vi "working_interface_timing.vi"(10 "VISA resource name":refnum<visa-resource-name>="TRIG") -> (2 "data in delay generator":dbl[](array[numeric]) caption="delay array" min=0.0 max=2000.0 format="%05.2f")   [LabVIEW 2011]
panel:
  out "timing write":u32
  in  "time unit":enum16{"s", "ms", "us", "ns"}(ring)=enum."us"
  in  "resolution":i32=100
  in  "duration":dbl[](array[numeric]) min=0.0 format="%.3f"
  in  "start time":dbl[](array[numeric]) format="%.3f"
  out "Digital Waveform Graph":digitalwaveform(graph)
  in  "write data":bool
  in  "read delay data":bool
  in  "stop":bool
  # "timing values are only relative,\n the absolute values are given in the\ndelay array!!!\n\nt0 and t can not be written to the device, t0 is always 0\nand  t is always the longest time + 25ns. However, t is \nused to display how long the nozzle is open to give a real \nrepresentation in the diagram (and only there). \nYou can change that time to pretty much any value, \nbut the nozzle itself is not controlled through the labview\n software. You have to set the time manually at the \nnozzle driver and ideally you should then enter that time\nfor t as well!\n\ndelay array index:\n0 - t0 = nozzle start (TTL) = 0\n1 - nozzle duration\n2 - power AMP START\n3 - power AMP STOP\n4 - AWG START (TTL)\n5 - AWG STOP (NA)\n6 - SWITCH ON \n7 - SWITCH OFF\n8 - OSC START (TTL)\n9 - OSC STOP (NA)\n\nTTL -> tool starts on rising flank\nof signal, hence the falling flank \nand the duration are not important!"
  # "t0 is always 0"
  # "AWG must start after power AMP is on \nand while it is still on!"
  # "SWITCH must NOT switch ON before \npower AMP is off!"
  # "delay array index:\n0 - to = nozzle start (TTL) = 0\n1 - t = nozzle duration\n2 - A = power AMP START\n3 - B = power AMP STOP\n4 - C = AWG START (TTL)\n5 - D = AWG STOP (NA)\n6 - E = SWITCH ON \n7 - F = SWITCH OFF\n8 - G = OSC START (TTL)\n9 - H = OSC STOP (NA)\n\nTTL -> tool starts on rising flank\nof signal, hence the falling flank \nand the duration are not important!"
  # "the graph does not show the actual TTL signal for all signals. For those with negative polarity it shows the inverse of the signal \nit shows when everything is active"
  # "nozzle"
  # "power AMP"
  # "AWG"
  # "SWITCH"
  # "OSC"
  # "t0"
  # "t"
  # "A"
  # "B"
  # "C"
  # "D"
  # "E"
  # "F"
  # "G"
  # "H"
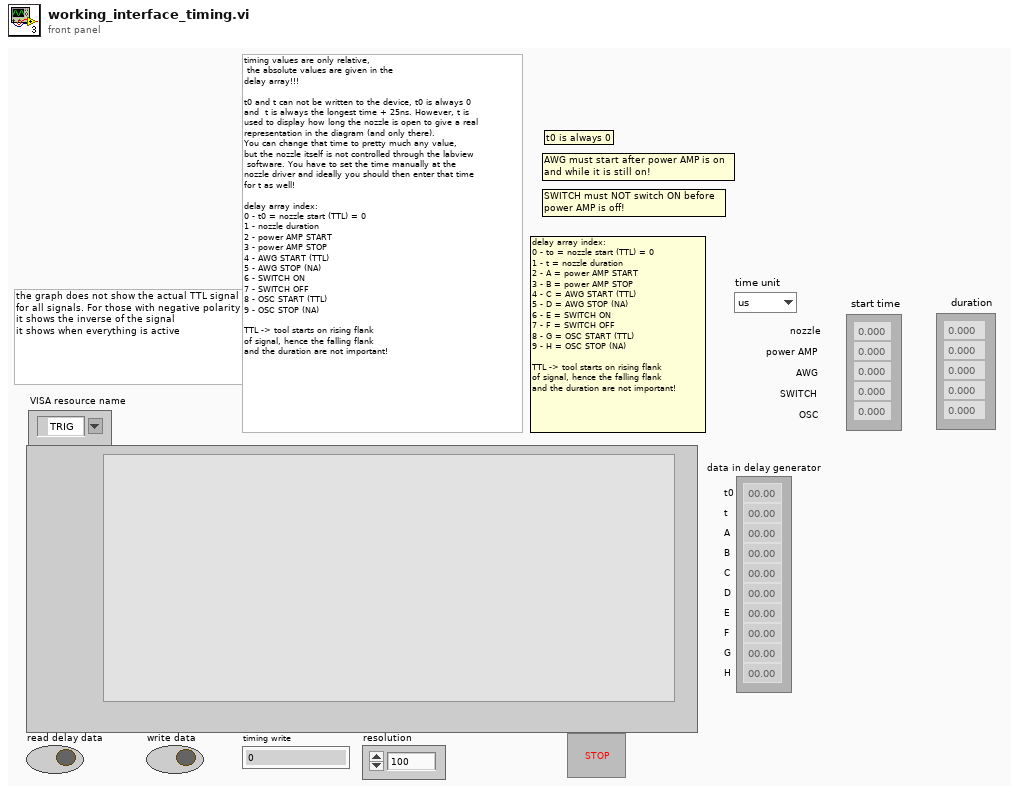
[diagram p1: front panel]
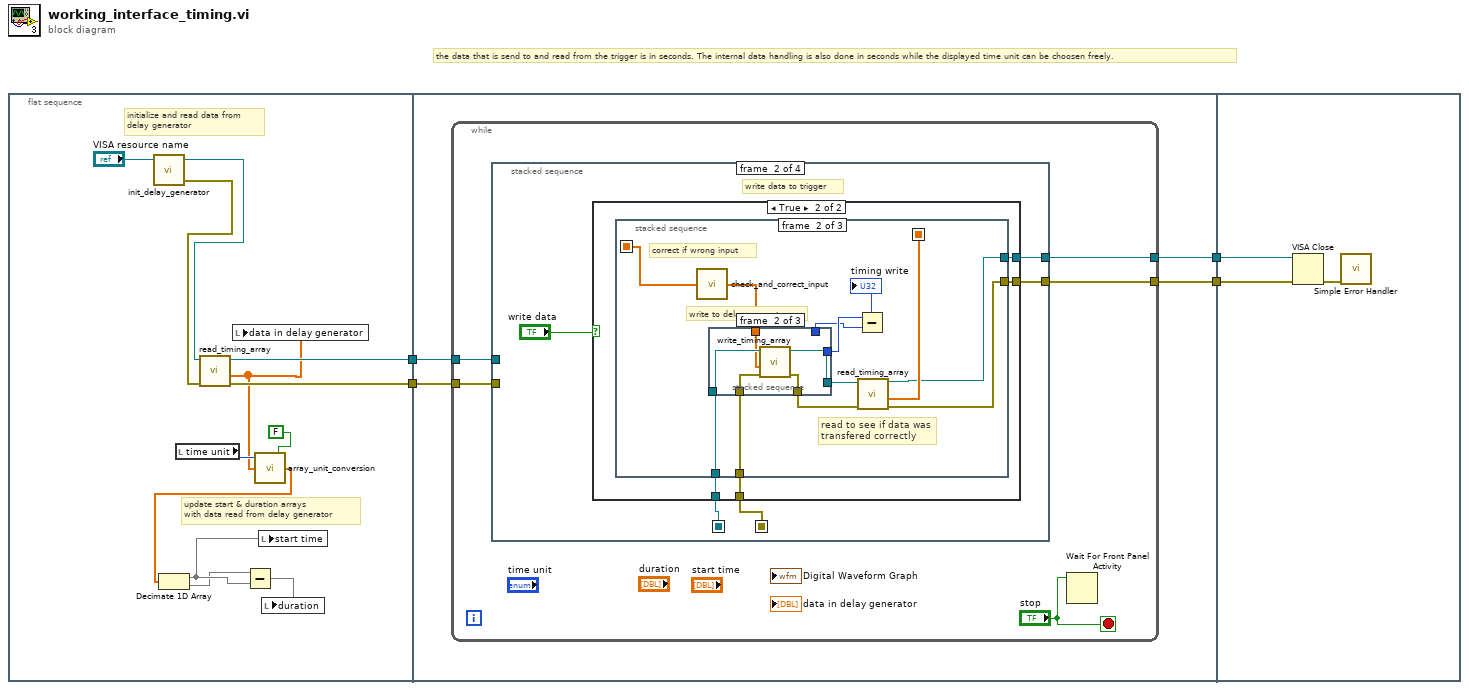
[diagram p0: block diagram]
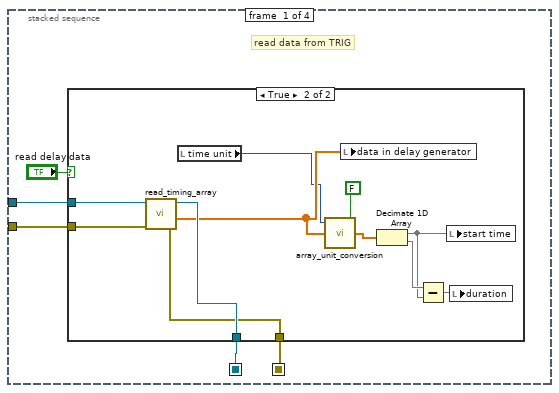
[diagram p2: hidden frame]
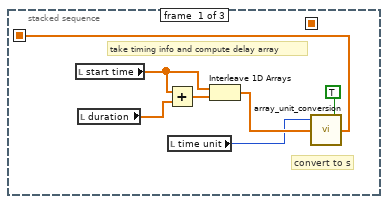
[diagram p5: hidden frame]
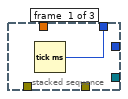
[diagram p6: hidden frame]
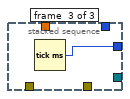
[diagram p7: hidden frame]
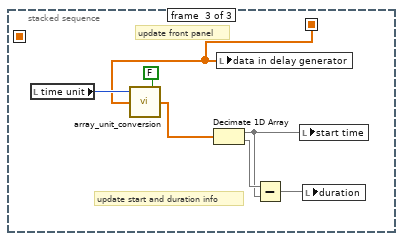
[diagram p8: hidden frame]
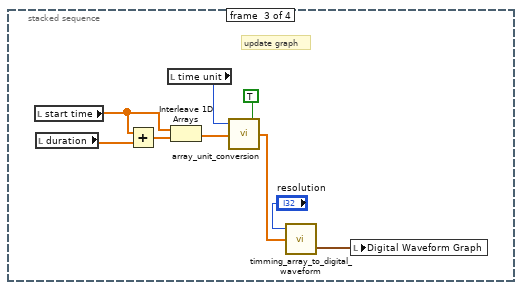
[diagram p9: hidden frame]
diagram:
  # "the data that is send to and read from the trigger is in seconds. The internal data handling is also done in seconds while the displayed time unit can be choosen freely."
  n1 = flat-sequence {
    tunnel: [w15] -> w4
    tunnel: [w16] -> w3
    tunnel: w4 -> [w20]
    tunnel: w3 -> [w19]
    tunnel: [w18] -> w2
    tunnel: [w17] -> w1
    tunnel: w2 -> [w99]
    tunnel: w1 -> [w98]
    frame #0 {
      # "update start & duration arrays \nwith data read from delay generator"
      # "initialize and read data from \ndelay generator"
      n2 = call "init_delay_generator.vi"("VISA resource name"="VISA resource name") -> ("error out"=w9:errorcluster, "VISA resource name out"=w10:refnum<visa-resource-name>)  [unwired: 3 in]
      n3 = local read "time unit"() -> (w8:enum16{"s", "ms", "us", "ns"})
      n4 = call "read_timing_array.vi"("error in"=w9, "VISA resource in"=w10) -> ("error out 2"=w16:errorcluster, "delay array"=w7:dbl[], "VISA resource out"=w15:refnum<visa-resource-name>)  [unwired: 3 in]
      n5 = local write "data in delay generator"(w7) -> ()
      n6 = call "array_unit_conversion.vi"("inverse function (arb. unit to s)?"=FALSE, "delay array"=w7, "time unit"=w8) -> ("output"=w6:dbl[])  [unwired: 2 in]
      n7 = Decimate 1D Array(w6) -> (w13:dbl[], w12:dbl[])
      n8 = Subtract(x=w12, y=w13) -> (x-y=w14:dbl[])
      n9 = local write "start time"(w13) -> ()
      n10 = local write "duration"(w14) -> ()
    }
    frame #1 {
      n11 = while {
        tunnel: w19 -> [w23]
        tunnel: [w25] -> w18
        tunnel: [w24] -> w17
        tunnel: w20 -> [w21]
        stop <- "stop" stop-if-true
        n12 = stacked-sequence {
          seq-local: [w28 _ _ _] -> [_ w47 _ _]
          seq-local: [w27 _ _ _] -> [_ w46 _ _]
          tunnel: w21 -> [w30 _ _ _]
          tunnel: w23 -> [w29 _ _ _]
          tunnel: [_ w44 _ _] -> w24
          tunnel: [_ w45 _ _] -> w25
          frame #0 {
            # "read data from TRIG"
            n13 = case shown="True" "read delay data" {
              tunnel: w30 -> [w31 w43]
              tunnel: w29 -> [w32 w42]
              tunnel: [w31 w41] -> w28
              tunnel: [w32 w40] -> w27
              frame False {
              }
              frame True {
                n14 = call "read_timing_array.vi"("error in"=w42, "VISA resource in"=w43) -> ("error out 2"=w40:errorcluster, "delay array"=w36:dbl[], "VISA resource out"=w41:refnum<visa-resource-name>)  [unwired: 3 in]
                n15 = local read "time unit"() -> (w35:enum16{"s", "ms", "us", "ns"})
                n16 = call "array_unit_conversion.vi"("inverse function (arb. unit to s)?"=FALSE, "delay array"=w36, "time unit"=w35) -> ("output"=w33:dbl[])  [unwired: 2 in]
                n17 = local write "data in delay generator"(w36) -> ()
                n18 = Decimate 1D Array(w33) -> (w37:dbl[], w38:dbl[])
                n19 = Subtract(x=w38, y=w37) -> (x-y=w39:dbl[])
                n20 = local write "start time"(w37) -> ()
                n21 = local write "duration"(w39) -> ()
              }
            }
          }
          frame #1 {
            # "write data to trigger"
            n22 = case shown="True" "write data" {
              tunnel: w47 -> [w49 w54]
              tunnel: w46 -> [w50 w53]
              tunnel: [w49 w52] -> w45
              tunnel: [w50 w51] -> w44
              frame False {
              }
              frame True {
                n23 = stacked-sequence {
                  seq-local: [w55 _ _] -> [_ w69 _]
                  seq-local: [_ w68 _] -> [_ _ w83]
                  tunnel: w54 -> [_ w73 _]
                  tunnel: w53 -> [_ w72 _]
                  tunnel: [_ w63 _] -> w52
                  tunnel: [_ w62 _] -> w51
                  frame #0 {
                    # "convert to s"
                    # "take timing info and compute delay array"
                    n24 = local read "start time"() -> (w60:dbl[])
                    n25 = local read "duration"() -> (w59:dbl[])
                    n26 = Add(x=w60, y=w59) -> (x+y=w61:dbl[])
                    n27 = local read "time unit"() -> (w56:enum16{"s", "ms", "us", "ns"})
                    n28 = Interleave 1D Arrays(w60, w61) -> (w57:dbl[])
                    n29 = call "array_unit_conversion.vi"("inverse function (arb. unit to s)?"=TRUE, "delay array"=w57, "time unit"=w56) -> ("output"=w55:dbl[])  [unwired: 2 in]
                  }
                  frame #1 {
                    # "read to see if data was \ntransfered correctly"
                    # "write to delay generator"
                    # "correct if wrong input"
                    n30 = call "check_and_correct_input.vi"("delay array"=w69) -> ("corrrected delay array"=w67:dbl[])  [unwired: 4 in]
                    n31 = stacked-sequence {
                      tunnel: w73 -> [_ w79 _]
                      tunnel: w72 -> [_ w78 _]
                      tunnel: [_ w77 _] -> w71
                      tunnel: [_ w76 _] -> w70
                      tunnel: w67 -> [_ w75 _]
                      tunnel: [w74 _ _] -> w64
                      tunnel: [_ _ w80] -> w65
                      frame #0 {
                        n32 = Tick Count (ms)() -> (millisecond timer value=w74:u32)
                      }
                      frame #1 {
                        n33 = call "write_timing_array.vi"("error in"=w78, "delay array"=w75, "VISA resource in"=w79) -> ("error out 2"=w76:errorcluster, "VISA resource out"=w77:refnum<visa-resource-name>)  [unwired: 2 in, 1 out]
                      }
                      frame #2 {
                        n34 = Tick Count (ms)() -> (millisecond timer value=w80:u32)
                      }
                    }
                    n35 = Subtract(x=w65, y=w64) -> (x-y=→"timing write":u32)
                    n36 = call "read_timing_array.vi"("error in"=w70, "VISA resource in"=w71) -> ("error out 2"=w62:errorcluster, "delay array"=w68:dbl[], "VISA resource out"=w63:refnum<visa-resource-name>)  [unwired: 3 in]
                  }
                  frame #2 {
                    # "update front panel"
                    # "update start and duration info"
                    n37 = local read "time unit"() -> (w84:enum16{"s", "ms", "us", "ns"})
                    n38 = call "array_unit_conversion.vi"("inverse function (arb. unit to s)?"=FALSE, "delay array"=w83, "time unit"=w84) -> ("output"=w82:dbl[])  [unwired: 2 in]
                    n39 = Decimate 1D Array(w82) -> (w85:dbl[], w87:dbl[])
                    n40 = local write "data in delay generator"(w83) -> ()
                    n41 = Subtract(x=w87, y=w85) -> (x-y=w86:dbl[])
                    n42 = local write "start time"(w85) -> ()
                    n43 = local write "duration"(w86) -> ()
                  }
                }
              }
            }
          }
          frame #2 {
            # "update graph"
            n44 = local read "start time"() -> (w90:dbl[])
            n45 = local read "duration"() -> (w89:dbl[])
            n46 = Add(x=w90, y=w89) -> (x+y=w94:dbl[])
            n47 = local read "time unit"() -> (w91:enum16{"s", "ms", "us", "ns"})
            n48 = Interleave 1D Arrays(w90, w94) -> (w92:dbl[])
            n49 = call "array_unit_conversion.vi"("inverse function (arb. unit to s)?"=TRUE, "delay array"=w92, "time unit"=w91) -> ("output"=w88:dbl[])  [unwired: 2 in]
            n50 = call "timming_array_to_digital_waveform.vi"("delay array"=w88, "resolution"="resolution") -> ("digital waveform"=w96:digitalwaveform)  [unwired: 2 in]
            n51 = local write "Digital Waveform Graph"(w96) -> ()
          }
          frame #3 {
            # "*RCL 3"
            # "*SAV 3"
          }
        }
        n52 = Wait For Front Panel Activity(3:"stop") -> ()  [unwired: 2 in, 1 out]
      }
    }
    frame #2 {
      n53 = VISA Close(VISA resource name=w99, error in (no error)=w98) -> (error out=w97:errorcluster)
      n54 = call <vilib>:"Simple Error Handler.vi"("error in (no error)"=w97) -> ()  [unwired: 4 in, 5 out]
    }
  }
